vi "Unsubscribe from Topic.vi"(8 "error in (no error)":errorcluster, 9 "Topic":string, 10 "Subscriber Enq":refnum<class "Message Enqueuer.lvclass">, 11 "Publisher in":refnum<class "Publisher.lvclass">) -> (0 "error out":errorcluster, 3 "Publisher out":refnum<class "Publisher.lvclass">)   [LabVIEW 2021, in "Publisher.lvclass"]
uses:
  Publisher.lvclass
  <vilib>/ActorFramework/Message Enqueuer/Message Enqueuer.lvclass
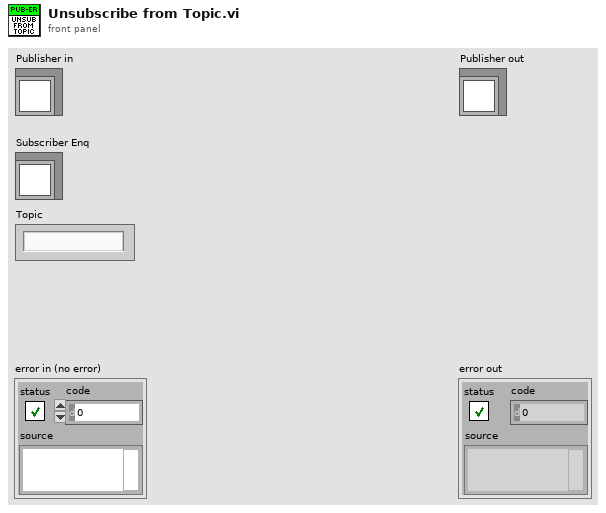
[diagram p1: front panel]
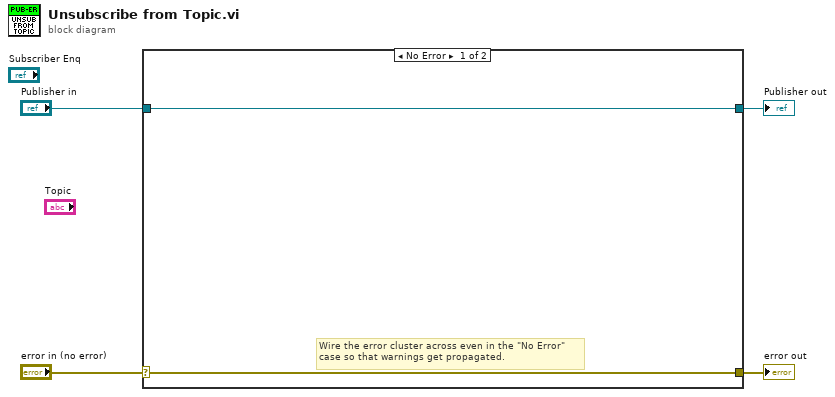
[diagram p0: block diagram]
diagram:
  n1 = case shown="No Error" "error in (no error)" {
    selector: "error in (no error)" -> [w5 w8]
    tunnel: [w5 w8] -> w3
    tunnel: [w6 w7] -> w1
    tunnel: "Publisher in" -> [w6 w7]
    frame No Error {
      # "Wire the error cluster across even in the \"No Error\"\ncase so that warnings get propagated."
    }
    frame Error {
    }
  }
  "error out" <- w3
  "Publisher out" <- w1
